vi "Initialise.vi"(8 "error in (no error)":errorcluster, 10 "Instrument Ref":string, 11 "Keysight 6700C in":refnum<class "Keysight 6700C.lvclass">) -> (0 "error out":errorcluster, 3 "Keysight 6700C out":refnum<class "Keysight 6700C.lvclass">)   [LabVIEW 2021, in "Concrete.lvlib" / "Keysight 6700C.lvclass"]
uses:
  Keysight 6700C.lvclass
  Keysight 6700C.lvclass/Keysight 6700C.ctl
  Harware Abstraction/AnalogIO/Power Supply.lvclass
  <instrlib>/Agilent N6700 Series/Agilent N6700 Series.lvlib
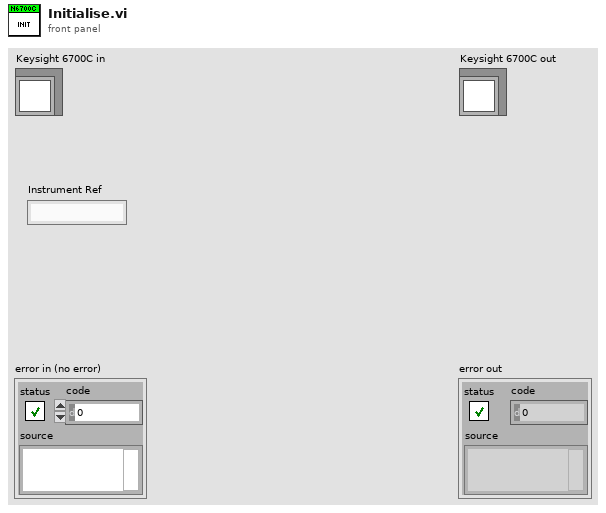
[diagram p1: front panel]
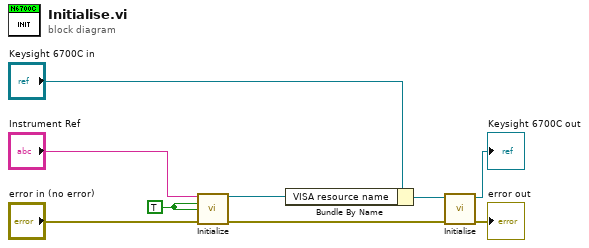
[diagram p0: block diagram]
diagram:
  w7 = TRUE ("Reset? (T: Yes)")
  n1 = call <instrlib>:"Initialize.vi"("VISA resource name"="Instrument Ref", "ID Query? (T: Yes)"=w7, "Reset? (T: Yes)"=w7, "error in (no error)"="error in (no error)") -> ("VISA resource name out"=w1:refnum<visa-resource-name>, "error out"=w5:errorcluster)  [unwired: 10 in]
  n2 = Bundle By Name(cluster="Keysight 6700C in", "VISA resource name"=w1) -> (w2:refnum<class "Keysight 6700C.lvclass">)
  n3 = call-parent "Initialise.vi"("error in (no error)"=w5, "Instrument in"=w2) -> ("error out"=→"error out":errorcluster, "Instrument out"=→"Keysight 6700C out":refnum<class "Keysight 6700C.lvclass">)  [unwired: 8 in]
